vi "nanocal -- nuclear schottky fit V3.vi"() -> ()   [LabVIEW 2020] (continued)
κ0\"-> 0.000000003681  , \"mm1\"-> 0.000000000000  , \"mm2\"-> 0.000000000000  , \"mm3\"-> 0.000000000000  , \"T\"->  0.512000000000  , \"B\"-> 12.000000000000  , \"θ\"-> 90.000000000000  |>   , \r8079 ->   <| \"ζ\"->  0.020568815513  , \"τ1\"-> 0.023045965648  , \"τS\"-> 0.020791387386  , \"τN\"-> 0.002229171297  , \"τC\"-> 0.004427475438  , \"κ0\"-> 0.000000004398  , \"mm1\"-> 0.000000000000  , \"mm2\"-> 0.000000000000  , \"mm3\"-> 0.000000000000  , \"T\"->  0.610000000000  , \"B\"-> 12.000000000000  , \"θ\"-> 90.000000000000  |>   , \r8080 ->   <| \"ζ\"->  0.016548170999  , \"τ1\"-> 0.020108887890  , \"τS\"-> 0.018558394948  , \"τN\"-> 0.001160732495  , \"τC\"-> 0.004746126241  , \"κ0\"-> 0.000000005882  , \"mm1\"-> 0.000000000000  , \"mm2\"-> 0.000000000000  , \"mm3\"-> 0.000000000000  , \"T\"->  0.810000000000  , \"B\"-> 12.000000000000  , \"θ\"-> 90.000000000000  |>   , \r8081 ->   <| \"ζ\"->  0.014495870556  , \"τ1\"-> 0.019990087457  , \"τS\"-> 0.016832201384  , \"τN\"-> 0.000455517238  , \"τC\"-> 0.005555782498  , \"κ0\"-> 0.000000008420  , \"mm1\"-> 0.000000000000  , \"mm2\"-> 0.000000000000  , \"mm3\"-> 0.000000000000  , \"T\"->  1.100000000000  , \"B\"-> 12.000000000000  , \"θ\"-> 90.000000000000  |>   , \r8082 ->   <| \"ζ\"->  0.014043763709  , \"τ1\"-> 0.018292068543  , \"τS\"-> 0.011311396743  , \"τN\"-> 0.000128802259  , \"τC\"-> 0.008087849636  , \"κ0\"-> 0.000000014258  , \"mm1\"-> 0.000000000000  , \"mm2\"-> 0.000000000000  , \"mm3\"-> 0.000000000000  , \"T\"->  1.800000000000  , \"B\"-> 12.000000000000  , \"θ\"-> 90.000000000000  |>   , \r8083 ->   <| \"ζ\"->  0.016187684631  , \"τ1\"-> 0.018325345271  , \"τS\"-> 0.007510087776  , \"τN\"-> 0.000028419157  , \"τC\"-> 0.008115463080  , \"κ0\"-> 0.000000024747  , \"mm1\"-> 0.000000000000  , \"mm2\"-> 0.000000000000  , \"mm3\"-> 0.000000000000  , \"T\"->  3.000000000000  , \"B\"-> 12.000000000000  , \"θ\"-> 90.000000000000  |>   , \r8084 ->   <| \"ζ\"->  0.027897403691  , \"τ1\"-> 0.014639690770  , \"τS\"-> 0.004105291179  , \"τN\"-> 0.000006999171  , \"τC\"-> 0.007414449545  , \"κ0\"-> 0.000000059701  , \"mm1\"-> 0.000000000000  , \"mm2\"-> 0.000000000000  , \"mm3\"-> 0.000000000000  , \"T\"->  5.700000000000  , \"B\"-> 12.000000000000  , \"θ\"-> 90.000000000000  |>   , \r8094 ->   <| \"ζ\"->  0.000000000000  , \"τ1\"-> 0.000000000000  , \"τS\"-> 0.000000000000  , \"τN\"-> 0.000000000000  , \"τC\"-> 0.000000000000  , \"κ0\"-> 0.000000000000  , \"mm1\"-> 0.000000000000  , \"mm2\"-> 0.000000000000  , \"mm3\"-> 0.000000000000  , \"T\"->  0.300000000000  , \"B\"-> 6.000000000000  , \"θ\"-> 90.000000000000  |>   , \r8095 ->   <| \"ζ\"->  0.132901556203  , \"τ1\"-> 0.022795175616  , \"τS\"-> 0.082481385864  , \"τN\"-> 0.041432545456  , \"τC\"-> 0.001408424074  , \"κ0\"-> 0.000000001182  , \"mm1\"-> 0.000000000000  , \"mm2\"-> 0.000000000000  , \"mm3\"-> 0.000000000000  , \"T\"->  0.197000000000  , \"B\"-> 6.000000000000  , \"θ\"-> 90.000000000000  |>   , \r8098 ->   <| \"ζ\"->  0.000000000000  , \"τ1\"-> 0.000000000000  , \"τS\"-> 0.000000000000  , \"τN\"-> 0.000000000000  , \"τC\"-> 0.000000000000  , \"κ0\"-> 0.000000000000  , \"mm1\"-> 0.000000000000  , \"mm2\"-> 0.000000000000  , \"mm3\"-> 0.000000000000  , \"T\"->  0.148000000000  , \"B\"-> 6.000000000000  , \"θ\"-> 90.000000000000  |>   , \r8099 ->   <| \"ζ\"->  0.132534999612  , \"τ1\"-> 0.042581417401  , \"τS\"-> 0.054103824371  , \"τN\"-> 0.072163013930  , \"τC\"-> 0.001421040158  , \"κ0\"-> 0.000000001190  , \"mm1\"-> 0.000000000000  , \"mm2\"-> 0.000000000000  , \"mm3\"-> 0.000000000000  , \"T\"->  0.197000000000  , \"B\"-> 9.000000000000  , \"θ\"-> 90.000000000000  |>   , \r8100 ->   <| \"ζ\"->  0.124414912597  , \"τ1\"-> 0.052685716706  , \"τS\"-> 0.041788480794  , \"τN\"-> 0.092820346766  , \"τC\"-> 0.001183564004  , \"κ0\"-> 0.000000001217  , \"mm1\"-> 0.000000000000  , \"mm2\"-> 0.000000000000  , \"mm3\"-> 0.000000000000  , \"T\"->  0.197000000000  , \"B\"-> 11.000000000000  , \"θ\"-> 90.000000000000  |>   , \r8101 ->   <| \"ζ\"->  0.130083148284  , \"τ1\"-> 0.046211117525  , \"τS\"-> 0.046173592526  , \"τN\"-> 0.081942172735  , \"τC\"-> 0.001380184863  , \"κ0\"-> 0.000000001209  , \"mm1\"-> 0.000000000000  , \"mm2\"-> 0.000000000000  , \"mm3\"-> 0.000000000000  , \"T\"->  0.197000000000  , \"B\"-> 10.000000000000  , \"θ\"-> 90.000000000000  |>   , \r8102 ->   <| \"ζ\"->  0.126440702434  , \"τ1\"-> 0.034118036572  , \"τS\"-> 0.060921114440  , \"τN\"-> 0.059832148427  , \"τC\"-> 0.001404471084  , \"κ0\"-> 0.000000001199  , \"mm1\"-> 0.000000000000  , \"mm2\"-> 0.000000000000  , \"mm3\"-> 0.000000000000  , \"T\"->  0.197000000000  , \"B\"-> 8.000000000000  , \"θ\"-> 90.000000000000  |>   , \r8103 ->   <| \"ζ\"->  0.131383255045  , \"τ1\"-> 0.026827335842  , \"τS\"-> 0.071725959535  , \"τN\"-> 0.047510049318  , \"τC\"-> 0.001407613780  , \"κ0\"-> 0.000000001187  , \"mm1\"-> 0.000000000000  , \"mm2\"-> 0.000000000000  , \"mm3\"-> 0.000000000000  , \"T\"->  0.197000000000  , \"B\"-> 7.000000000000  , \"θ\"-> 90.000000000000  |>   , \r8104 ->   <| \"ζ\"->  0.125455081262  , \"τ1\"-> 0.021777951907  , \"τS\"-> 0.089086097551  , \"τN\"-> 0.033580911935  , \"τC\"-> 0.001437991682  , \"κ0\"-> 0.000000001167  , \"mm1\"-> 0.000000000000  , \"mm2\"-> 0.000000000000  , \"mm3\"-> 0.000000000000  , \"T\"->  0.197000000000  , \"B\"-> 5.000000000000  , \"θ\"-> 90.000000000000  |>   , \r8105 ->   <| \"ζ\"->  0.101804363109  , \"τ1\"-> 0.031947692776  , \"τS\"-> 0.014125667853  , \"τN\"-> 0.006009042128  , \"τC\"-> 0.002323789932  , \"κ0\"-> 0.000000001168  , \"mm1\"-> 0.000000000000  , \"mm2\"-> 0.000000000000  , \"mm3\"-> 0.000000000000  , \"T\"->  0.197000000000  , \"B\"-> 0.000000000000  , \"θ\"-> 90.000000000000  |>   , \r8106 ->   <| \"ζ\"->  0.000000000000  , \"τ1\"-> 0.000000000000  , \"τS\"-> 0.000000000000  , \"τN\"-> 0.000000000000  , \"τC\"-> 0.000000000000  , \"κ0\"-> 0.000000000000  , \"mm1\"-> 0.000000000000  , \"mm2\"-> 0.000000000000  , \"mm3\"-> 0.000000000000  , \"T\"->  1.550000000000  , \"B\"-> 0.000000000000  , \"θ\"-> 90.000000000000  |>   , \r8107 ->   <| \"ζ\"->  0.000000000000  , \"τ1\"-> 0.000000000000  , \"τS\"-> 0.000000000000  , \"τN\"-> 0.000000000000  , \"τC\"-> 0.000000000000  , \"κ0\"-> 0.000000000000  , \"mm1\"-> 0.000000000000  , \"mm2\"-> 0.000000000000  , \"mm3\"-> 0.000000000000  , \"T\"->  1.000000000000  , \"B\"-> 0.000000000000  , \"θ\"-> 90.000000000000  |>   , \r8108 ->   <| \"ζ\"->  0.000000000000  , \"τ1\"-> 0.000000000000  , \"τS\"-> 0.000000000000  , \"τN\"-> 0.000000000000  , \"τC\"-> 0.000000000000  , \"κ0\"-> 0.000000000000  , \"mm1\"-> 0.000000000000  , \"mm2\"-> 0.000000000000  , \"mm3\"-> 0.000000000000  , \"T\"->  0.670000000000  , \"B\"-> 0.000000000000  , \"θ\"-> 90.000000000000  |>   , \r8110 ->   <| \"ζ\"->  0.162585495535  , \"τ1\"-> 0.037883389730  , \"τS\"-> 0.086562863191  , \"τN\"-> 0.241872534356  , \"τC\"-> 0.001506143871  , \"κ0\"-> 0.000000000791  , \"mm1\"-> 0.000000000000  , \"mm2\"-> 0.000000000000  , \"mm3\"-> 0.000000000000  , \"T\"->  0.160000000000  , \"B\"-> 12.000000000000  , \"θ\"-> 30.000000000000  |>   , \r8112 ->   <| \"ζ\"->  0.156472219566  , \"τ1\"-> 0.031017925061  , \"τS\"-> 0.080872234530  , \"τN\"-> 0.219381306397  , \"τC\"-> 0.001437792153  , \"κ0\"-> 0.000000000867  , \"mm1\"-> 0.000000000000  , \"mm2\"-> 0.000000000000  , \"mm3\"-> 0.000000000000  , \"T\"->  0.170000000000  , \"B\"-> 12.000000000000  , \"θ\"-> 30.000000000000  |>   , \r8113 ->   <| \"ζ\"->  0.211545693132  , \"τ1\"-> 0.029106147473  , \"τS\"-> 0.094475691604  , \"τN\"-> 0.369151052631  , \"τC\"-> 0.001396700790  , \"κ0\"-> 0.000000000537  , \"mm1\"-> 0.000000000000  , \"mm2\"-> 0.000000000000  , \"mm3\"-> 0.000000000000  , \"T\"->  0.140000000000  , \"B\"-> 12.000000000000  , \"θ\"-> 30.000000000000  |>   , \r8114 ->   <| \"ζ\"->  0.128615765969  , \"τ1\"-> 0.032665502211  , \"τS\"-> 0.082694869013  , \"τN\"-> 0.105788373632  , \"τC\"-> 0.001439686784  , \"κ0\"-> 0.000000001168  , \"mm1\"-> 0.000000000000  , \"mm2\"-> 0.000000000000  , \"mm3\"-> 0.000000000000  , \"T\"->  0.200000000000  , \"B\"-> 12.000000000000  , \"θ\"-> 30.000000000000  |>   , \r8115 ->   <| \"ζ\"->  0.072634365939  , \"τ1\"-> 0.028637109000  , \"τS\"-> 0.065061142288  , \"τN\"-> 0.040304243071  , \"τC\"-> 0.001622979999  , \"κ0\"-> 0.000000001498  , \"mm1\"-> 0.000000000000  , \"mm2\"-> 0.000000000000  , \"mm3\"-> 0.000000000000  , \"T\"->  0.250000000000  , \"B\"-> 12.000000000000  , \"θ\"-> 30.000000000000  |>   , \r8116 ->   <| \"ζ\"->  0.050663808076  , \"τ1\"-> 0.024940898568  , \"τS\"-> 0.056803871413  , \"τN\"-> 0.018856862265  , \"τC\"-> 0.002133501904  , \"κ0\"-> 0.000000001888  , \"mm1\"-> 0.000000000000  , \"mm2\"-> 0.000000000000  , \"mm3\"-> 0.000000000000  , \"T\"->  0.300000000000  , \"B\"-> 12.000000000000  , \"θ\"-> 30.000000000000  |>   , \r8117 ->   <| \"ζ\"->  0.036420486357  , \"τ1\"-> 0.020986681106  , \"τS\"-> 0.049149577509  , \"τN\"-> 0.011109585503  , \"τC\"-> 0.002819780093  , \"κ0\"-> 0.000000002299  , \"mm1\"-> 0.000000000000  , \"mm2\"-> 0.000000000000  , \"mm3\"-> 0.000000000000  , \"T\"->  0.360000000000  , \"B\"-> 12.000000000000  , \"θ\"-> 30.000000000000  |>   , \r8118 ->   <| \"ζ\"->  0.028468689077  , \"τ1\"-> 0.020220821810  , \"τS\"-> 0.043529484347  , \"τN\"-> 0.005653540941  , \"τC\"-> 0.003150537442  , \"κ0\"-> 0.000000002855  , \"mm1\"-> 0.000000000000  , \"mm2\"-> 0.000000000000  , \"mm3\"-> 0.000000000000  , \"T\"->  0.430000000000  , \"B\"-> 12.000000000000  , \"θ\"-> 30.000000000000  |>   , \r8119 ->   <| \"ζ\"->  0.021116250068  , \"τ1\"-> 0.020669239851  , \"τS\"-> 0.037941648749  , \"τN\"-> 0.003221866945  , \"τC\"-> 0.003619427775  , \"κ0\"-> 0.000000003553  , \"mm1\"-> 0.000000000000  , \"mm2\"-> 0.000000000000  , \"mm3\"-> 0.000000000000  , \"T\"->  0.530000000000  , \"B\"-> 12.000000000000  , \"θ\"-> 30.000000000000  |>   , \r8120 ->   <| \"ζ\"->  0.016892016292  , \"τ1\"-> 0.020344757415  , \"τS\"-> 0.033845756966  , \"τN\"-> 0.001946817417  , \"τC\"-> 0.004013762913  , \"κ0\"-> 0.000000004252  , \"mm1\"-> 0.000000000000  , \"mm2\"-> 0.000000000000  , \"mm3\"-> 0.000000000000  , \"T\"->  0.620000000000  , \"B\"-> 12.000000000000  , \"θ\"-> 30.000000000000  |>   , \r8121 ->   <| \"ζ\"->  0.013460153434  , \"τ1\"-> 0.020684726260  , \"τS\"-> 0.027140346721  , \"τN\"-> 0.000960302406  , \"τC\"-> 0.004517434882  , \"κ0\"-> 0.000000005889  , \"mm1\"-> 0.000000000000  , \"mm2\"-> 0.000000000000  , \"mm3\"-> 0.000000000000  , \"T\"->  0.830000000000  , \"B\"-> 12.000000000000  , \"θ\"-> 30.000000000000  |>   , \r8122 ->   <| \"ζ\"->  0.010912011148  , \"τ1\"-> 0.020760977312  , \"τS\"-> 0.021106239637  , \"τN\"-> 0.000452316988  , \"τC\"-> 0.005003723454  , \"κ0\"-> 0.000000008194  , \"mm1\"-> 0.000000000000  , \"mm2\"-> 0.000000000000  , \"mm3\"-> 0.000000000000  , \"T\"->  1.130000000000  , \"B\"-> 12.000000000000  , \"θ\"-> 30.000000000000  |>   , \r8123 ->   <| \"ζ\"->  0.009772435939  , \"τ1\"-> 0.020827345370  , \"τS\"-> 0.013809334085  , \"τN\"-> 0.000168485133  , \"τC\"-> 0.005555066716  , \"κ0\"-> 0.000000013930  , \"mm1\"-> 0.000000000000  , \"mm2\"-> 0.000000000000  , \"mm3\"-> 0.000000000000  , \"T\"->  1.900000000000  , \"B\"-> 12.000000000000  , \"θ\"-> 30.000000000000  |>   , \r8124 ->   <| \"ζ\"->  0.010111127240  , \"τ1\"-> 0.020788755574  , \"τS\"-> 0.009968978424  , \"τN\"-> 0.000077788811  , \"τC\"-> 0.004598584548  , \"κ0\"-> 0.000000024346  , \"mm1\"-> 0.000000000000  , \"mm2\"-> 0.000000000000  , \"mm3\"-> 0.000000000000  , \"T\"->  3.100000000000  , \"B\"-> 12.000000000000  , \"θ\"-> 30.000000000000  |>   , \r40047 ->   <| \"ζ\"->  0.020744689680  , \"τ1\"-> 0.017944253087  , \"τS\"-> 0.003548154619  , \"τN\"-> 0.000036329906  , \"τC\"-> 0.004738266852  , \"κ0\"-> 0.000000058027  , \"mm1\"-> 0.000000000000  , \"mm2\"-> 0.000000000000  , \"mm3\"-> 0.000000000000  , \"T\"->  19.600000000000  , \"B\"-> 12.000000000000  , \"θ\"-> 60.000000000000  |>   , \r40049 ->   <| \"ζ\"->  0.334519022578  , \"τ1\"-> 0.071617660141  , \"τS\"-> 0.066230384072  , \"τN\"-> 0.374518999658  , \"τC\"-> 0.002158821958  , \"κ0\"-> 0.000000000405  , \"mm1\"-> 0.000000000000  , \"mm2\"-> 0.000000000000  , \"mm3\"-> 0.000000000000  , \"T\"->  0.129000000000  , \"B\"-> 12.000000000000  , \"θ\"-> 60.000000000000  |>   , \r40125 ->   <| \"ζ\"->  0.295520923520  , \"τ1\"-> 0.054772440405  , \"τS\"-> 0.071814005451  , \"τN\"-> 0.249593767169  , \"τC\"-> 0.001103632155  , \"κ0\"-> 0.000000000625  , \"mm1\"-> 0.000000000000  , \"mm2\"-> 0.000000000000  , \"mm3\"-> 0.000000000000  , \"T\"->  0.157000000000  , \"B\"-> 12.000000000000  , \"θ\"-> 45.000000000000  |>   , \r40126 ->   <| \"ζ\"->  0.523545279740  , \"τ1\"-> 0.065613539167  , \"τS\"-> 0.100000000000  , \"τN\"-> 0.424083114177  , \"τC\"-> 0.000911255863  , \"κ0\"-> 0.000000000418  , \"mm1\"-> 0.000000000000  , \"mm2\"-> 0.000000000000  , \"mm3\"-> 0.000000000000  , \"T\"->  0.120000000000  , \"B\"-> 12.000000000000  , \"θ\"-> 45.000000000000  |>   , \r40127 ->   <| \"ζ\"->  0.273742116471  , \"τ1\"-> 0.052262909995  , \"τS\"-> 0.060554036646  , \"τN\"-> 0.154269705680  , \"τC\"-> 0.001074144337  , \"κ0\"-> 0.000000000753  , \"mm1\"-> 0.000000000000  , \"mm2\"-> 0.000000000000  , \"mm3\"-> 0.000000000000  , \"T\"->  0.170000000000  , \"B\"-> 12.000000000000  , \"θ\"-> 45.000000000000  |>   , \r40128 ->   <| \"ζ\"->  0.215688135788  , \"τ1\"-> 0.043710888546  , \"τS\"-> 0.044756474141  , \"τN\"-> 0.090222547904  , \"τC\"-> 0.001049781785  , \"κ0\"-> 0.000000001047  , \"mm1\"-> 0.000000000000  , \"mm2\"-> 0.000000000000  , \"mm3\"-> 0.000000000000  , \"T\"->  0.200000000000  , \"B\"-> 12.000000000000  , \"θ\"-> 45.000000000000  |>   , \r40129 ->   <| \"ζ\"->  0.118583992968  , \"τ1\"-> 0.035232851003  , \"τS\"-> 0.037458022816  , \"τN\"-> 0.033724509363  , \"τC\"-> 0.001440922263  , \"κ0\"-> 0.000000001360  , \"mm1\"-> 0.000000000000  , \"mm2\"-> 0.000000000000  , \"mm3\"-> 0.000000000000  , \"T\"->  0.255000000000  , \"B\"-> 12.000000000000  , \"θ\"-> 45.000000000000  |>   , \r40130 ->   <| \"ζ\"->  0.085152769414  , \"τ1\"-> 0.029001116263  , \"τS\"-> 0.032604663993  , \"τN\"-> 0.016878763935  , \"τC\"-> 0.001443524845  , \"κ0\"-> 0.000000001728  , \"mm1\"-> 0.000000000000  , \"mm2\"-> 0.000000000000  , \"mm3\"-> 0.000000000000  , \"T\"->  0.300000000000  , \"B\"-> 12.000000000000  , \"θ\"-> 45.000000000000  |>   , \r40131 ->   <| \"ζ\"->  0.061011838044  , \"τ1\"-> 0.025440548989  , \"τS\"-> 0.030028053978  , \"τN\"-> 0.010140731955  , \"τC\"-> 0.001895079687  , \"κ0\"-> 0.000000002115  , \"mm1\"-> 0.000000000000  , \"mm2\"-> 0.000000000000  , \"mm3\"-> 0.000000000000  , \"T\"->  0.360000000000  , \"B\"-> 12.000000000000  , \"θ\"-> 45.000000000000  |>   , \r40132 ->   <| \"ζ\"->  0.046686299518  , \"τ1\"-> 0.021011215626  , \"τS\"-> 0.027633142317  , \"τN\"-> 0.005348477555  , \"τC\"-> 0.002098477650  , \"κ0\"-> 0.000000002635  , \"mm1\"-> 0.000000000000  , \"mm2\"-> 0.000000000000  , \"mm3\"-> 0.000000000000  , \"T\"->  0.430000000000  , \"B\"-> 12.000000000000  , \"θ\"-> 45.000000000000  |>   , \r40133 ->   <| \"ζ\"->  0.035204330012  , \"τ1\"-> 0.021011523093  , \"τS\"-> 0.025247316079  , \"τN\"-> 0.002718647875  , \"τC\"-> 0.003091727575  , \"κ0\"-> 0.000000003296  , \"mm1\"-> 0.000000000000  , \"mm2\"-> 0.000000000000  , \"mm3\"-> 0.000000000000  , \"T\"->  0.530000000000  , \"B\"-> 12.000000000000  , \"θ\"-> 45.000000000000  |>   , \r40134 ->   <| \"ζ\"->  0.030862035723  , \"τ1\"-> 0.019328530751  , \"τS\"-> 0.023568572597  , \"τN\"-> 0.001701966614  , \"τC\"-> 0.003453790534  , \"κ0\"-> 0.000000003906  , \"mm1\"-> 0.000000000000  , \"mm2\"-> 0.000000000000  , \"mm3\"-> 0.000000000000  , \"T\"->  0.620000000000  , \"B\"-> 12.000000000000  , \"θ\"-> 45.000000000000  |>   , \r40135 ->   <| \"ζ\"->  0.023591124045  , \"τ1\"-> 0.014910006225  , \"τS\"-> 0.019342950404  , \"τN\"-> 0.000752972387  , \"τC\"-> 0.004900413232  , \"κ0\"-> 0.000000005453  , \"mm1\"-> 0.000000000000  , \"mm2\"-> 0.000000000000  , \"mm3\"-> 0.000000000000  , \"T\"->  0.830000000000  , \"B\"-> 12.000000000000  , \"θ\"-> 45.000000000000  |>   , \r40136 ->   <| \"ζ\"->  0.020215154826  , \"τ1\"-> 0.014105227254  , \"τS\"-> 0.015660924043  , \"τN\"-> 0.000525137036  , \"τC\"-> 0.005447728357  , \"κ0\"-> 0.000000007594  , \"mm1\"-> 0.000000000000  , \"mm2\"-> 0.000000000000  , \"mm3\"-> 0.000000000000  , \"T\"->  1.130000000000  , \"B\"-> 12.000000000000  , \"θ\"-> 45.000000000000  |>   , \r40137 ->   <| \"ζ\"->  0.018090572724  , \"τ1\"-> 0.013314780956  , \"τS\"-> 0.010820835010  , \"τN\"-> 0.000265552167  , \"τC\"-> 0.005393540417  , \"κ0\"-> 0.000000013100  , \"mm1\"-> 0.000000000000  , \"mm2\"-> 0.000000000000  , \"mm3\"-> 0.000000000000  , \"T\"->  1.900000000000  , \"B\"-> 12.000000000000  , \"θ\"-> 45.000000000000  |>   , \r40138 ->   <| \"ζ\"->  0.019438138135  , \"τ1\"-> 0.013521019406  , \"τS\"-> 0.007253169401  , \"τN\"-> 0.000154824830  , \"τC\"-> 0.004746579385  , \"κ0\"-> 0.000000023466  , \"mm1\"-> 0.000000000000  , \"mm2\"-> 0.000000000000  , \"mm3\"-> 0.000000000000  , \"T\"->  3.100000000000  , \"B\"-> 12.000000000000  , \"θ\"-> 45.000000000000  |>   , \r40139 ->   <| \"ζ\"->  0.018573189054  , \"τ1\"-> 0.013304612245  , \"τS\"-> 0.003723860844  , \"τN\"-> 0.000084829442  , \"τC\"-> 0.004309703632  , \"κ0\"-> 0.000000058362  , \"mm1\"-> 0.000000000000  , \"mm2\"-> 0.000000000000  , \"mm3\"-> 0.000000000000  , \"T\"->  5.700000000000  , \"B\"-> 12.000000000000  , \"θ\"-> 45.000000000000  |>   , \r80047 ->   <| \"ζ\"->  0.000000000000  , \"τ1\"-> 0.000000000000  , \"τS\"-> 0.000000000000  , \"τN\"-> 0.000000000000  , \"τC\"-> 0.000000000000  , \"κ0\"-> 0.000000000000  , \"mm1\"-> 0.000000000000  , \"mm2\"-> 0.000000000000  , \"mm3\"-> 0.000000000000  , \"T\"->  19.600000000000  , \"B\"-> 12.000000000000  , \"θ\"-> 60.000000000000  |>   , \r80049 ->   <| \"ζ\"->  0.206128000000  , \"τ1\"-> 0.061001000000  , \"τS\"-> 0.056065000000  , \"τN\"-> 0.442324169403  , \"τC\"-> 0.001917000000  , \"κ0\"-> 0.000000000541  , \"mm1\"-> 0.000000000000  , \"mm2\"-> 0.000000000000  , \"mm3\"-> 0.000000000000  , \"T\"->  0.129000000000  , \"B\"-> 12.000000000000  , \"θ\"-> 60.000000000000  |>   , \r80125 ->   <| \"ζ\"->  0.000000000000  , \"τ1\"-> 0.000000000000  , \"τS\"-> 0.000000000000  , \"τN\"-> 0.000000000000  , \"τC\"-> 0.000000000000  , \"κ0\"-> 0.000000000000  , \"mm1\"-> 0.000000000000  , \"mm2\"-> 0.000000000000  , \"mm3\"-> 0.000000000000  , \"T\"->  0.157000000000  , \"B\"-> 12.000000000000  , \"θ\"-> 45.000000000000  |>   , \r80126 ->   <| \"ζ\"->  0.000000000000  , \"τ1\"-> 0.000000000000  , \"τS\"-> 0.000000000000  , \"τN\"-> 0.000000000000  , \"τC\"-> 0.000000000000  , \"κ0\"-> 0.000000000000  , \"mm1\"-> 0.000000000000  , \"mm2\"-> 0.000000000000  , \"mm3\"-> 0.000000000000  , \"T\"->  0.120000000000  , \"B\"-> 12.000000000000  , \"θ\"-> 45.000000000000  |>   , \r80127 ->   <| \"ζ\"->  0.000000000000  , \"τ1\"-> 0.000000000000  , \"τS\"-> 0.000000000000  , \"τN\"-> 0.000000000000  , \"τC\"-> 0.000000000000  , \"κ0\"-> 0.000000000000  , \"mm1\"-> 0.000000000000  , \"mm2\"-> 0.000000000000  , \"mm3\"-> 0.000000000000  , \"T\"->  0.170000000000  , \"B\"-> 12.000000000000  , \"θ\"-> 45.000000000000  |>   , \r80128 ->   <| \"ζ\"->  0.000000000000  , \"τ1\"-> 0.000000000000  , \"τS\"-> 0.000000000000  , \"τN\"-> 0.000000000000  , \"τC\"-> 0.000000000000  , \"κ0\"-> 0.000000000000  , \"mm1\"-> 0.000000000000  , \"mm2\"-> 0.000000000000  , \"mm3\"-> 0.000000000000  , \"T\"->  0.200000000000  , \"B\"-> 12.000000000000  , \"θ\"-> 45.000000000000  |>   , \r80129 ->   <| \"ζ\"->  0.000000000000  , \"τ1\"-> 0.000000000000  , \"τS\"-> 0.000000000000  , \"τN\"-> 0.000000000000  , \"τC\"-> 0.000000000000  , \"κ0\"-> 0.000000000000  , \"mm1\"-> 0.000000000000  , \"mm2\"-> 0.000000000000  , \"mm3\"-> 0.000000000000  , \"T\"->  0.255000000000  , \"B\"-> 12.000000000000  , \"θ\"-> 45.000000000000  |>   , \r80130 ->   <| \"ζ\"->  0.000000000000  , \"τ1\"-> 0.000000000000  , \"τS\"-> 0.000000000000  , \"τN\"-> 0.000000000000  , \"τC\"-> 0.000000000000  , \"κ0\"-> 0.000000000000  , \"mm1\"-> 0.000000000000  , \"mm2\"-> 0.000000000000  , \"mm3\"-> 0.000000000000  , \"T\"->  0.300000000000  , \"B\"-> 12.000000000000  , \"θ\"-> 45.000000000000  |>   , \r80131 ->   <| \"ζ\"->  0.000000000000  , \"τ1\"-> 0.000000000000  , \"τS\"-> 0.000000000000  , \"τN\"-> 0.000000000000  , \"τC\"-> 0.000000000000  , \"κ0\"-> 0.000000000000  , \"mm1\"-> 0.000000000000  , \"mm2\"-> 0.000000000000  , \"mm3\"-> 0.000000000000  , \"T\"->  0.360000000000  , \"B\"-> 12.000000000000  , \"θ\"-> 45.000000000000  |>   , \r80132 ->   <| \"ζ\"->  0.000000000000  , \"τ1\"-> 0.000000000000  , \"τS\"-> 0.000000000000  , \"τN\"-> 0.000000000000  , \"τC\"-> 0.000000000000  , \"κ0\"-> 0.000000000000  , \"mm1\"-> 0.000000000000  , \"mm2\"-> 0.000000000000  , \"mm3\"-> 0.000000000000  , \"T\"->  0.430000000000  , \"B\"-> 12.000000000000  , \"θ\"-> 45.000000000000  |>   , \r80133 ->   <| \"ζ\"->  0.000000000000  , \"τ1\"-> 0.000000000000  , \"τS\"-> 0.000000000000  , \"τN\"-> 0.000000000000  , \"τC\"-> 0.000000000000  , \"κ0\"-> 0.000000000000  , \"mm1\"-> 0.000000000000  , \"mm2\"-> 0.000000000000  , \"mm3\"-> 0.000000000000  , \"T\"->  0.530000000000  , \"B\"-> 12.000000000000  , \"θ\"-> 45.000000000000  |>   , \r80134 ->   <| \"ζ\"->  0.000000000000  , \"τ1\"-> 0.000000000000  , \"τS\"-> 0.000000000000  , \"τN\"-> 0.000000000000  , \"τC\"-> 0.000000000000  , \"κ0\"-> 0.000000000000  , \"mm1\"-> 0.000000000000  , \"mm2\"-> 0.000000000000  , \"mm3\"-> 0.000000000000  , \"T\"->  0.620000000000  , \"B\"-> 12.000000000000  , \"θ\"-> 45.000000000000  |>   , \r80135 ->   <| \"ζ\"->  0.000000000000  , \"τ1\"-> 0.000000000000  , \"τS\"-> 0.000000000000  , \"τN\"-> 0.000000000000  , \"τC\"-> 0.000000000000  , \"κ0\"-> 0.000000000000  , \"mm1\"-> 0.000000000000  , \"mm2\"-> 0.000000000000  , \"mm3\"-> 0.000000000000  , \"T\"->  0.830000000000  , \"B\"-> 12.000000000000  , \"θ\"-> 45.000000000000  |>   , \r80136 ->   <| \"ζ\"->  0.000000000000  , \"τ1\"-> 0.000000000000  , \"τS\"-> 0.000000000000  , \"τN\"-> 0.000000000000  , \"τC\"-> 0.000000000000  , \"κ0\"-> 0.000000000000  , \"mm1\"-> 0.000000000000  , \"mm2\"-> 0.000000000000  , \"mm3\"-> 0.000000000000  , \"T\"->  1.130000000000  , \"B\"-> 12.000000000000  , \"θ\"-> 45.000000000000  |>   , \r80137 ->   <| \"ζ\"->  0.000000000000  , \"τ1\"-> 0.000000000000  , \"τS\"-> 0.000000000000  , \"τN\"-> 0.000000000000  , \"τC\"-> 0.000000000000  , \"κ0\"-> 0.000000000000  , \"mm1\"-> 0.000000000000  , \"mm2\"-> 0.000000000000  , \"mm3\"-> 0.000000000000  , \"T\"->  1.900000000000  , \"B\"-> 12.000000000000  , \"θ\"-> 45.000000000000  |>   , \r80138 ->   <| \"ζ\"->  0.000000000000  , \"τ1\"-> 0.000000000000  , \"τS\"-> 0.000000000000  , \"τN\"-> 0.000000000000  , \"τC\"-> 0.000000000000  , \"κ0\"-> 0.000000000000  , \"mm1\"-> 0.000000000000  , \"mm2\"-> 0.000000000000  , \"mm3\"-> 0.000000000000  , \"T\"->  3.100000000000  , \"B\"-> 12.000000000000  , \"θ\"-> 45.000000000000  |>   , \r80139 ->   <| \"ζ\"->  0.000000000000  , \"τ1\"-> 0.000000000000  , \"τS\"-> 0.000000000000  , \"τN\"-> 0.000000000000  , \"τC\"-> 0.000000000000  , \"κ0\"-> 0.000000000000  , \"mm1\"-> 0.000000000000  , \"mm2\"-> 0.000000000000  , \"mm3\"-> 0.000000000000  , \"T\"->  5.700000000000  , \"B\"-> 12.000000000000  , \"θ\"-> 45.000000000000  |>   , \r"
  in  "Math --> string OUT!":bool
  in  "string IN  --> Math!":bool
  in  "file pattern":string="CeCoIn5_*_labview_.dat"
  in  "folder":path=path "/opt/new/Dropbox/shared_AkashAndreas/paper-CeCoIn5/dataset--changeT--12T--0deg--60deg--90deg"
  in  "filenames":u16(ring)=29 caption="files" items=["CeCoIn5_2nd_8047_12T_sam_0.12K_0deg_changeT_fsweep_labview_.dat", "CeCoIn5_2nd_8071_12T_sam_0.120K_90deg_changeT_fsweep_labview_.dat", "CeCoIn5_4th___40126__(040)__C(f)_12T_0.120K_45deg_changeT_ref_fromraw__labview_.dat", "CeCoIn5_4th___80126__(040)__C(f)_12T_0.120K_45deg_changeT_sam_fromraw__labview_.dat", "CeCoIn5_3rd_4026_ref_12T_0.127K_60deg_changeT_fsweep_labview_.dat", "CeCoIn5_3rd_8026_sam_12T_0.127K_60deg_changeT_fsweep_labview_.dat", "CeCoIn5_3rd_40049_ref_12T_0.129K_60deg_changeT_fsweep_labview_.dat", "CeCoIn5_3rd_80049_sam_12T_0.129K_60deg_changeT_fsweep_labview_.dat", "CeCoIn5_2nd_4047_12T_ref_0.14K_0deg_changeT_fsweep_labview_.dat", "CeCoIn5_2nd_4071_12T_ref_0.14K_90deg_changeT_fsweep_labview_.dat", "CeCoIn5_4th_4113_ref_12T_0.14K_30deg_changeT_fsweep_labview_.dat", "CeCoIn5_4th_8113_sam_12T_0.14K_30deg_changeT_fsweep_labview_.dat", "CeCoIn5_2nd_4098_6T_0.148K_90deg_ref_changeB_fsweep_labview_.dat", "CeCoIn5_2nd_8048_12T_sam_0.148K_0deg_changeT_fsweep_labview_.dat", "CeCoIn5_2nd_8072_12T_sam_0.148K_90deg_changeT_fsweep_labview_.dat", "CeCoIn5_2nd_8098_6T_0.148K_90deg_sam_changeB_fsweep_labview_.dat", "CeCoIn5_3rd_4027_ref_12T_0.15K_60deg_changeT_fsweep_labview_.dat", "CeCoIn5_3rd_8027_sam_12T_0.15K_60deg_changeT_fsweep_labview_.dat", "CeCoIn5_4th___40125__(039)__C(f)_12T_0.157K_45deg _changeT_ref_fromraw__labview_.dat", "CeCoIn5_4th___80125__(039)__C(f)_12T_0.157K_45deg _changeT_sam_fromraw__labview_.dat", "CeCoIn5_4th_4110_ref_12T_0.16K_30deg_changeT_fsweep_labview_.dat", "CeCoIn5_4th_8110_sam_12T_0.16K_30deg_changeT_fsweep_labview_.dat", "CeCoIn5_2nd_4048_12T_ref_0.17K_0deg_changeT_fsweep_labview_.dat", "CeCoIn5_4th_4112_ref_12T_0.17K_30deg_changeT_fsweep_labview_.dat", "CeCoIn5_4th_8112_sam_12T_0.17K_30deg_changeT_fsweep_labview_.dat", "CeCoIn5_4th___40127__(041)__C(f)_12T_0.170K_45deg_changeT_ref_fromraw__labview_.dat", "CeCoIn5_4th___80127__(041)__C(f)_12T_0.170K_45deg_changeT_sam_fromraw__labview_.dat", "CeCoIn5_3rd_4028_ref_12T_0.179K_60deg_changeT_fsweep_labview_.dat", "CeCoIn5_3rd_8028_sam_12T_0.179K_60deg_changeT_fsweep_labview_.dat", "CeCoIn5_2nd_8049_12T_sam_0.179K_0deg_changeT_fsweep_labview_.dat", "CeCoIn5_2nd_8070_12T_sam_0.179K_90deg_changeT_fsweep_labview_.dat", "CeCoIn5_2nd_4072_12T_ref_0.18K_90deg_changeT_fsweep_labview_.dat", "CeCoIn5_2nd_4095_6T_0.197K_90deg_ref_changeB_fsweep_labview_.dat", "CeCoIn5_2nd_4099_9T_0.197K_90deg_ref_changeB_fsweep_labview_.dat", "CeCoIn5_2nd_4100_11T_0.197K_90deg_ref_changeB_fsweep_labview_.dat", "CeCoIn5_2nd_4101_10T_0.197K_90deg_ref_changeB_fsweep_labview_.dat", "CeCoIn5_2nd_4102_8T_0.197K_90deg_ref_changeB_fsweep_labview_.dat", "CeCoIn5_2nd_4103_7T_0.197K_90deg_ref_changeB_fsweep_labview_.dat", "CeCoIn5_2nd_4104_5T_0.197K_90deg_ref_changeB_fsweep_labview_.dat", "CeCoIn5_2nd_4105_0T_0.197K_90deg_ref_changeB_fsweep_labview_.dat", "CeCoIn5_2nd_8050_12T_sam_0.197K_0deg_changeT_fsweep_labview_.dat", "CeCoIn5_2nd_8073_12T_sam_0.197K_90deg_changeT_fsweep_labview_.dat", "CeCoIn5_2nd_8095_6T_0.197K_90deg_sam_changeB_fsweep_labview_.dat", "CeCoIn5_2nd_8099_9T_0.197K_90deg_sam_changeB_fsweep_labview_.dat", "CeCoIn5_2nd_8100_11T_0.197K_90deg_sam_changeB_fsweep_labview_.dat", "CeCoIn5_2nd_8101_10T_0.197K_90deg_sam_changeB_fsweep_labview_.dat", "CeCoIn5_2nd_8102_8T_0.197K_90deg_sam_changeB_fsweep_labview_.dat", "CeCoIn5_2nd_8103_7T_0.197K_90deg_sam_changeB_fsweep_labview_.dat", "CeCoIn5_2nd_8104_5T_0.197K_90deg_sam_changeB_fsweep_labview_.dat", "CeCoIn5_2nd_8105_0T_0.197K_90deg_sam_changeB_fsweep_labview_.dat", "CeCoIn5_3rd_4029_ref_12T_0.20K_60deg_changeT_fsweep_labview_.dat", "CeCoIn5_2nd_4049_12T_ref_0.20K_0deg_changeT_fsweep_labview_.dat", "CeCoIn5_2nd_4070_12T_ref_0.20K_90deg_changeT_fsweep_labview_.dat", "CeCoIn5_4th_4114_ref_12T_0.20K_30deg_changeT_fsweep_labview_.dat", "CeCoIn5_3rd_8029_sam_12T_0.20K_60deg_changeT_fsweep_labview_.dat", "CeCoIn5_4th_8114_sam_12T_0.20K_30deg_changeT_fsweep_labview_.dat", "CeCoIn5_4th___40128__(042)__C(f)_12T_0.200K_45deg_changeT_ref_fromraw__labview_.dat", "CeCoIn5_4th___80128__(042)__C(f)_12T_0.200K_45deg_changeT_sam_fromraw__labview_.dat", "CeCoIn5_2nd_4050_12T_ref_0.22K_0deg_changeT_fsweep_labview_.dat", "CeCoIn5_2nd_4073_12T_ref_0.22K_90deg_changeT_fsweep_labview_.dat", "CeCoIn5_3rd_4030_ref_12T_0.24K_60deg_changeT_fsweep_labview_.dat", "CeCoIn5_3rd_8030_sam_12T_0.24K_60deg_changeT_fsweep_labview_.dat", "CeCoIn5_2nd_8074_12T_sam_0.249K_90deg_changeT_fsweep_labview_.dat", "CeCoIn5_4th_4115_ref_12T_0.25K_30deg_changeT_fsweep_labview_.dat", "CeCoIn5_2nd_8051_12T_sam_0.25K_0deg_changeT_fsweep_labview_.dat", "CeCoIn5_4th_8115_sam_12T_0.25K_30deg_changeT_fsweep_labview_.dat", "CeCoIn5_4th___40129__(043)__C(f)_12T_0.255K_45deg_changeT_ref_fromraw__labview_.dat", "CeCoIn5_4th___80129__(043)__C(f)_12T_0.255K_45deg_changeT_sam_fromraw__labview_.dat", "CeCoIn5_2nd_4074_12T_ref_0.27K_90deg_changeT_fsweep_labview_.dat", "CeCoIn5_2nd_4051_12T_ref_0.28K_0deg_changeT_fsweep_labview_.dat", "CeCoIn5_3rd_4031_ref_12T_0.287K_60deg_changeT_fsweep_labview_.dat", "CeCoIn5_3rd_8031_sam_12T_0.287K_60deg_changeT_fsweep_labview_.dat", "CeCoIn5_2nd_4094_6T_0.30K_90deg_ref_changeB_fsweep_labview_.dat", "CeCoIn5_4th_4116_ref_12T_0.30K_30deg_changeT_fsweep_labview_.dat", "CeCoIn5_2nd_8052_12T_sam_0.3K_0deg_changeT_fsweep_labview_.dat", "CeCoIn5_2nd_8075_12T_sam_0.300K_90deg_changeT_fsweep_labview_.dat", "CeCoIn5_2nd_8094_6T_0.30K_90deg_sam_changeB_fsweep_labview_.dat", "CeCoIn5_4th_8116_sam_12T_0.30K_30deg_changeT_fsweep_labview_.dat", "CeCoIn5_4th___40130__(044)__C(f)_12T_0.300K_45deg_changeT_ref_fromraw__labview_.dat", "CeCoIn5_4th___80130__(044)__C(f)_12T_0.300K_45deg_changeT_sam_fromraw__labview_.dat", "CeCoIn5_3rd_4032_ref_12T_0.33K_60deg_changeT_fsweep_labview_.dat", "CeCoIn5_2nd_4052_12T_ref_0.33K_0deg_changeT_fsweep_labview_.dat", "CeCoIn5_2nd_4075_12T_ref_0.33K_90deg_changeT_fsweep_labview_.dat", "CeCoIn5_3rd_8032_sam_12T_0.33K_60deg_changeT_fsweep_labview_.dat", "CeCoIn5_4th_4117_ref_12T_0.36K_30deg_changeT_fsweep_labview_.dat", "CeCoIn5_2nd_8053_12T_sam_0.360K_0deg_changeT_fsweep_labview_.dat", "CeCoIn5_2nd_8076_12T_sam_0.360K_90deg_changeT_fsweep_labview_.dat", "CeCoIn5_4th_8117_sam_12T_0.36K_30deg_changeT_fsweep_labview_.dat", "CeCoIn5_4th___40131__(045)__C(f)_12T_0.360K_45deg_changeT_ref_fromraw__labview_.dat", "CeCoIn5_4th___80131__(045)__C(f)_12T_0.360K_45deg_changeT_sam_fromraw__labview_.dat", "CeCoIn5_2nd_4076_12T_ref_0.39K_90deg_changeT_fsweep_labview_.dat", "CeCoIn5_2nd_4053_12T_ref_0.40K_0deg_changeT_fsweep_labview_.dat", "CeCoIn5_3rd_4033_ref_12T_0.43K_60deg_changeT_fsweep_labview_.dat", "CeCoIn5_4th_4118_ref_12T_0.43K_30deg_changeT_fsweep_labview_.dat", "CeCoIn5_3rd_8033_sam_12T_0.43K_60deg_changeT_fsweep_labview_.dat", "CeCoIn5_2nd_8054_12T_sam_0.430K_0deg_changeT_fsweep_labview_.dat", "CeCoIn5_2nd_8077_12T_sam_0.430K_90deg_changeT_fsweep_labview_.dat", "CeCoIn5_4th_8118_sam_12T_0.43K_30deg_changeT_fsweep_labview_.dat", "CeCoIn5_4th___40132__(046)__C(f)_12T_0.43K_45deg_changeT_ref_fromraw__labview_.dat", "CeCoIn5_4th___80132__(046)__C(f)_12T_0.43K_45deg_changeT_sam_fromraw__labview_.dat", "CeCoIn5_2nd_4054_12T_ref_0.48K_0deg_changeT_fsweep_labview_.dat", "CeCoIn5_2nd_4077_12T_ref_0.48K_90deg_changeT_fsweep_labview_.dat", "CeCoIn5_3rd_4034_ref_12T_0.51K_60deg_changeT_fsweep_labview_.dat", "CeCoIn5_3rd_8034_sam_12T_0.51K_60deg_changeT_fsweep_labview_.dat", "CeCoIn5_2nd_8055_12T_sam_0.512K_0deg_changeT_fsweep_labview_.dat", "CeCoIn5_2nd_8078_12T_sam_0.512K_90deg_changeT_fsweep_labview_.dat", "CeCoIn5_4th_4119_ref_12T_0.53K_30deg_changeT_fsweep_labview_.dat", "CeCoIn5_4th_8119_sam_12T_0.53K_30deg_changeT_fsweep_labview_.dat", "CeCoIn5_4th___40133__(047)__C(f)_12T_0.53K_45deg_changeT_ref_fromraw__labview_.dat", "CeCoIn5_4th___80133__(047)__C(f)_12T_0.53K_45deg_changeT_sam_fromraw__labview_.dat", "CeCoIn5_2nd_4055_12T_ref_0.58K_0deg_changeT_fsweep_labview_.dat", "CeCoIn5_2nd_4078_12T_ref_0.58K_90deg_changeT_fsweep_labview_.dat", "CeCoIn5_2nd_8056_12T_sam_0.61K_0deg_changeT_fsweep_labview_.dat", "CeCoIn5_2nd_8079_12T_sam_0.610K_90deg_changeT_fsweep_labview_.dat", "CeCoIn5_3rd_4035_ref_12T_0.62K_60deg_changeT_fsweep_labview_.dat", "CeCoIn5_4th_4120_ref_12T_0.62K_30deg_changeT_fsweep_labview_.dat", "CeCoIn5_3rd_8035_sam_12T_0.62K_60deg_changeT_fsweep_labview_.dat", "CeCoIn5_4th_8120_sam_12T_0.62K_30deg_changeT_fsweep_labview_.dat", "CeCoIn5_4th___40134__(048)__C(f)_12T_0.62K_45deg_changeT_ref_fromraw__labview_.dat", "CeCoIn5_4th___80134__(048)__C(f)_12T_0.62K_45deg_changeT_sam_fromraw__labview_.dat", "CeCoIn5_2nd_4108_0T_0.67K_90deg_ref_changeB_fsweep_labview_.dat", "CeCoIn5_2nd_8108_0T_0.67K_90deg_sam_changeB_fsweep_labview_.dat", "CeCoIn5_2nd_4056_12T_ref_0.68K_0deg_changeT_fsweep_labview_.dat", "CeCoIn5_2nd_4079_12T_ref_0.68K_90deg_changeT_fsweep_labview_.dat", "CeCoIn5_2nd_8057_12T_sam_0.81K_0deg_changeT_fsweep_labview_.dat", "CeCoIn5_2nd_8080_12T_sam_0.810K_90deg_changeT_fsweep_labview_.dat", "CeCoIn5_3rd_4036_ref_12T_0.83K_60deg_changeT_fsweep_labview_.dat", "CeCoIn5_4th_4121_ref_12T_0.83K_30deg_changeT_fsweep_labview_.dat", "CeCoIn5_3rd_8036_sam_12T_0.83K_60deg_changeT_fsweep_labview_.dat", "CeCoIn5_4th_8121_sam_12T_0.83K_30deg_changeT_fsweep_labview_.dat", "CeCoIn5_4th___40135__(049)__C(f)_12T_0.83K_45deg_changeT_ref_fromraw__labview_.dat", "CeCoIn5_4th___80135__(049)__C(f)_12T_0.83K_45deg_changeT_sam_fromraw__labview_.dat", "CeCoIn5_2nd_4057_12T_ref_0.91K_0deg_changeT_fsweep_labview_.dat", "CeCoIn5_2nd_4080_12T_ref_0.91K_90deg_changeT_fsweep_labview_.dat", "CeCoIn5_2nd_4107_0T_1.00K_90deg_ref_changeB_fsweep_labview_.dat", "CeCoIn5_2nd_8107_0T_1.00K_90deg_sam_changeB_fsweep_labview_.dat", "CeCoIn5_2nd_8081_12T_sam_1.1K_90deg_changeT_fsweep_labview_.dat", "CeCoIn5_2nd_8058_12T_sam_1.12K_0deg_changeT_fsweep_labview_.dat", "CeCoIn5_3rd_4037_ref_12T_1.13K_60deg_changeT_fsweep_labview_.dat", "CeCoIn5_4th_4122_ref_12T_1.13K_30deg_changeT_fsweep_labview_.dat", "CeCoIn5_3rd_8037_sam_12T_1.13K_60deg_changeT_fsweep_labview_.dat", "CeCoIn5_4th_8122_sam_12T_1.13K_30deg_changeT_fsweep_labview_.dat", "CeCoIn5_4th___40136__(050)__C(f)_12T_1.13K_45deg_changeT_ref_fromraw__labview_.dat", "CeCoIn5_4th___80136__(050)__C(f)_12T_1.13K_45deg_changeT_sam_fromraw__labview_.dat", "CeCoIn5_2nd_4058_12T_ref_1.23K_0deg_changeT_fsweep_labview_.dat", "CeCoIn5_2nd_4081_12T_ref_1.23K_90deg_changeT_fsweep_labview_.dat", "CeCoIn5_2nd_4106_0T_1.55K_90deg_ref_changeB_fsweep_labview_.dat", "CeCoIn5_2nd_8106_0T_1.55K_90deg_sam_changeB_fsweep_labview_.dat", "CeCoIn5_2nd_8059_12T_sam_1.8K_0deg_changeT_fsweep_labview_.dat", "CeCoIn5_2nd_8082_12T_sam_1.8K_90deg_changeT_fsweep_labview_.dat", "CeCoIn5_3rd_4038_ref_12T_1.90K_60deg_changeT_fsweep_labview_.dat", "CeCoIn5_4th_4123_ref_12T_1.90K_30deg_changeT_fsweep_labview_.dat", "CeCoIn5_3rd_8038_sam_12T_1.90K_60deg_changeT_fsweep_labview_.dat", "CeCoIn5_4th_8123_sam_12T_1.90K_30deg_changeT_fsweep_labview_.dat", "CeCoIn5_4th___40137__(051)__C(f)_12T_1.90K_45deg_changeT_ref_fromraw__labview_.dat", "CeCoIn5_4th___80137__(051)__C(f)_12T_1.90K_45deg_changeT_sam_fromraw__labview_.dat", "CeCoIn5_2nd_4059_12T_ref_1.97K_0deg_changeT_fsweep_labview_.dat", "CeCoIn5_2nd_4082_12T_ref_2.05K_90deg_changeT_fsweep_labview_.dat", "CeCoIn5_2nd_8060_12T_sam_3.0K_0deg_changeT_fsweep_labview_.dat", "CeCoIn5_2nd_8083_12T_sam_3.0K_90deg_changeT_fsweep_labview_.dat", "CeCoIn5_4th_4124_ref_12T_3.10K_30deg_changeT_fsweep_labview_.dat", "CeCoIn5_4th_8124_sam_12T_3.10K_30deg_changeT_fsweep_labview_.dat", "CeCoIn5_4th___40138__(052)__C(f)_12T_3.10K_45deg_changeT_ref_fromraw__labview_.dat", "CeCoIn5_4th___80138__(052)__C(f)_12T_3.10K_45deg_changeT_sam_fromraw__labview_.dat", "CeCoIn5_3rd_4039_ref_12T_3.15K_60deg_changeT_fsweep_labview_.dat", "CeCoIn5_3rd_8039_sam_12T_3.15K_60deg_changeT_fsweep_labview_.dat", "CeCoIn5_2nd_4060_12T_ref_3.19K_0deg_changeT_fsweep_labview_.dat", "CeCoIn5_2nd_4083_12T_ref_3.31K_90deg_changeT_fsweep_labview_.dat", "CeCoIn5_2nd_8061_12T_sam_5.5K_0deg_changeT_fsweep_labview_.dat", "CeCoIn5_3rd_4040_ref_12T_5.70K_60deg_changeT_fsweep_labview_.dat", "CeCoIn5_3rd_8040_sam_12T_5.70K_60deg_changeT_fsweep_labview_.dat", "CeCoIn5_2nd_8084_12T_sam_5.7K_90deg_changeT_fsweep_labview_.dat", "CeCoIn5_4th___40139__(053)__C(f)_12T_5.70K_45deg_changeT_ref_fromraw__labview_.dat", "CeCoIn5_4th___80139__(053)__C(f)_12T_5.70K_45deg_changeT_sam_fromraw__labview_.dat", "CeCoIn5_2nd_4061_12T_ref_5.82K_0deg_changeT_fsweep_labview_.dat", "CeCoIn5_2nd_4084_12T_ref_6.0K_90deg_changeT_fsweep_labview_.dat", "CeCoIn5_3rd_4041_ref_12T_7.87K_60deg_changeT_fsweep_labview_.dat", "CeCoIn5_3rd_8041_sam_12T_7.87K_60deg_changeT_fsweep_labview_.dat", "CeCoIn5_3rd_4042_ref_12T_9.80K_60deg_changeT_fsweep_labview_.dat", "CeCoIn5_3rd_8042_sam_12T_9.80K_60deg_changeT_fsweep_labview_.dat", "CeCoIn5_3rd_4043_ref_12T_12.36K_60deg_changeT_fsweep_labview_.dat", "CeCoIn5_3rd_8043_sam_12T_12.36K_60deg_changeT_fsweep_labview_.dat", "CeCoIn5_3rd_4044_ref_12T_14.80K_60deg_changeT_fsweep_labview_.dat", "CeCoIn5_3rd_8044_sam_12T_14.80K_60deg_changeT_fsweep_labview_.dat", "CeCoIn5_3rd_4045_ref_12T_16.42K_60deg_changeT_fsweep_labview_.dat", "CeCoIn5_3rd_8045_sam_12T_16.42K_60deg_changeT_fsweep_labview_.dat", "CeCoIn5_3rd_4046_ref_12T_18.04K_60deg_changeT_fsweep_labview_.dat", "CeCoIn5_3rd_8046_sam_12T_18.04K_60deg_changeT_fsweep_labview_.dat", "CeCoIn5_3rd_40047_ref_12T_19.60K_60deg_changeT_fsweep_labview_.dat", "CeCoIn5_3rd_80047_sam_12T_19.60K_60deg_changeT_fsweep_labview_.dat"]
  out "notes":string="------------\n\n/opt/new/Dropbox/desktop_data/Indium-nanocal-cell12-June2021/labview-ready-files\nIndium_June2021_*_ark.dat\n\n---------------------\n/opt/new/Dropbox/shared_AkashAndreas/paper-CeCoIn5/labviewreadydata\nCeCoIn5_*_labview_.dat\n--------------------------------\n\n  48 ->   <| \"ζ\"->  0.219100303741  , \"τ1\"-> 0.028643012604  , \"τS\"-> 0.279362928811  , \"τN\"-> 0.246156444058  , \"τC\"-> 0.001272401549  , \"κ0\"-> 0.000000000760  , \"mm1\"-> 0.000227975653  , \"mm2\"-> 0.014929571562  , \"mm3\"-> 0.655418694024  , \"T\"->  0.148000000000  , \"B\"-> 12.000000000000  , \"θ\"-> 0.000000000000  |>   , \r49 ->   <| \"ζ\"->  0.172530402516  , \"τ1\"-> 0.028151242536  , \"τS\"-> 0.147833386881  , \"τN\"-> 0.151615465647  , \"τC\"-> 0.001078987959  , \"κ0\"-> 0.000000001040  , \"mm1\"-> 0.000157922197  , \"mm2\"-> 0.013374167913  , \"mm3\"-> 0.366811023972  , \"T\"->  0.179000000000  , \"B\"-> 12.000000000000  , \"θ\"-> 0.000000000000  |>   , \r50 ->   <| \"ζ\"->  0.133463068512  , \"τ1\"-> 0.025720252342  , \"τS\"-> 0.123146502099  , \"τN\"-> 0.097478248186  , \"τC\"-> 0.001335222055  , \"κ0\"-> 0.000000001204  , \"mm1\"-> 0.000155896243  , \"mm2\"-> 0.013755191011  , \"mm3\"-> 0.263214393590  , \"T\"->  0.197000000000  , \"B\"-> 12.000000000000  , \"θ\"-> 0.000000000000  |>   , \r51 ->   <| \"ζ\"->  0.081993362741  , \"τ1\"-> 0.028064095915  , \"τS\"-> 0.091433392476  , \"τN\"-> 0.030443971714  , \"τC\"-> 0.001450504959  , \"κ0\"-> 0.000000001536  , \"mm1\"-> 0.000108446090  , \"mm2\"-> 0.019905820843  , \"mm3\"-> 0.141370833064  , \"T\"->  0.250000000000  , \"B\"-> 12.000000000000  , \"θ\"-> 0.000000000000  |>   , \r52 ->   <| \"ζ\"->  0.054088186012  , \"τ1\"-> 0.023838802615  , \"τS\"-> 0.069079396629  , \"τN\"-> 0.016435267456  , \"τC\"-> 0.002025071743  , \"κ0\"-> 0.000000001955  , \"mm1\"-> 0.000101234646  , \"mm2\"-> 0.018244822177  , \"mm3\"-> 0.097657814678  , \"T\"->  0.300000000000  , \"B\"-> 12.000000000000  , \"θ\"-> 0.000000000000  |>   , \r53 ->   <| \"ζ\"->  0.039314966212  , \"τ1\"-> 0.020712803909  , \"τS\"-> 0.055413767550  , \"τN\"-> 0.008474403424  , \"τC\"-> 0.002674063387  , \"κ0\"-> 0.000000002415  , \"mm1\"-> 0.000096818147  , \"mm2\"-> 0.017190811405  , \"mm3\"-> 0.072499170001  , \"T\"->  0.360000000000  , \"B\"-> 12.000000000000  , \"θ\"-> 0.000000000000  |>   , \r54 ->   <| \"ζ\"->  0.031945976845  , \"τ1\"-> 0.019000922826  , \"τS\"-> 0.045624146388  , \"τN\"-> 0.005314716063  , \"τC\"-> 0.002488383471  , \"κ0\"-> 0.000000002954  , \"mm1\"-> 0.000073272643  , \"mm2\"-> 0.016306894362  , \"mm3\"-> 0.057675293464  , \"T\"->  0.430000000000  , \"B\"-> 12.000000000000  , \"θ\"-> 0.000000000000  |>   , \r55 ->   <| \"ζ\"->  0.023031239946  , \"τ1\"-> 0.018268814012  , \"τS\"-> 0.037269400776  , \"τN\"-> 0.002696792890  , \"τC\"-> 0.003257395394  , \"κ0\"-> 0.000000003720  , \"mm1\"-> 0.000067670174  , \"mm2\"-> 0.016445281937  , \"mm3\"-> 0.045899921957  , \"T\"->  0.512000000000  , \"B\"-> 12.000000000000  , \"θ\"-> 0.000000000000  |>   , \r56 ->   <| \"ζ\"->  0.019920170845  , \"τ1\"-> 0.016368892412  , \"τS\"-> 0.030579536580  , \"τN\"-> 0.001736017565  , \"τC\"-> 0.004971418152  , \"κ0\"-> 0.000000004410  , \"mm1\"-> 0.000083939556  , \"mm2\"-> 0.015095997595  , \"mm3\"-> 0.039119658918  , \"T\"->  0.610000000000  , \"B\"-> 12.000000000000  , \"θ\"-> 0.000000000000  |>   , \r57 ->   <| \"ζ\"->  0.017558473054  , \"τ1\"-> 0.014545104284  , \"τS\"-> 0.022979681288  , \"τN\"-> 0.000840829385  , \"τC\"-> 0.005228030240  , \"κ0\"-> 0.000000006068  , \"mm1\"-> 0.000073916527  , \"mm2\"-> 0.013750428362  , \"mm3\"-> 0.030187552103  , \"T\"->  0.810000000000  , \"B\"-> 12.000000000000  , \"θ\"-> 0.000000000000  |>   , \r58 ->   <| \"ζ\"->  0.011916480594  , \"τ1\"-> 0.012551282481  , \"τS\"-> 0.018233218660  , \"τN\"-> 0.000345702746  , \"τC\"-> 0.004699451527  , \"κ0\"-> 0.000000008451  , \"mm1\"-> 0.000044190864  , \"mm2\"-> 0.012162820727  , \"mm3\"-> 0.023844039179  , \"T\"->  1.120000000000  , \"B\"-> 12.000000000000  , \"θ\"-> 0.000000000000  |>   , \r59 ->   <| \"ζ\"->  0.012831327568  , \"τ1\"-> 0.013315909415  , \"τS\"-> 0.012590836847  , \"τN\"-> 0.000065003013  , \"τC\"-> 0.005276356243  , \"κ0\"-> 0.000000013610  , \"mm1\"-> 0.000047406274  , \"mm2\"-> 0.013137605540  , \"mm3\"-> 0.018225484932  , \"T\"->  1.800000000000  , \"B\"-> 12.000000000000  , \"θ\"-> 0.000000000000  |>   , \r60 ->   <| \"ζ\"->  0.019774146838  , \"τ1\"-> 0.013257273421  , \"τS\"-> 0.007064131508  , \"τN\"-> 0.000028000819  , \"τC\"-> 0.006942241845  , \"κ0\"-> 0.000000023477  , \"mm1\"-> 0.000068886863  , \"mm2\"-> 0.012935419574  , \"mm3\"-> 0.014427582022  , \"T\"->  3.000000000000  , \"B\"-> 12.000000000000  , \"θ\"-> 0.000000000000  |>   , \r61 ->   <| \"ζ\"->  0.029251354442  , \"τ1\"-> 0.014634751206  , \"τS\"-> 0.003873958746  , \"τN\"-> 0.000007000487  , \"τC\"-> 0.006827504775  , \"κ0\"-> 0.000000056438  , \"mm1\"-> 0.000072018576  , \"mm2\"-> 0.010723236476  , \"mm3\"-> 0.014661483476  , \"T\"->  5.500000000000  , \"B\"-> 12.000000000000  , \"θ\"-> 0.000000000000  |>   , \r70 ->   <| \"ζ\"->  0.166131699293  , \"τ1\"-> 0.072775930308  , \"τS\"-> 0.042465819987  , \"τN\"-> 0.161702990281  , \"τC\"-> 0.001278548133  , \"κ0\"-> 0.000000001029  , \"mm1\"-> 0.000178150965  , \"mm2\"-> 0.012296129795  , \"mm3\"-> 0.299667919341  , \"T\"->  0.179000000000  , \"B\"-> 12.000000000000  , \"θ\"-> 90.000000000000  |>   , \r71 ->   <| \"ζ\"->  0.300863384227  , \"τ1\"-> 0.104924004009  , \"τS\"-> 0.071070599729  , \"τN\"-> 0.992887187112  , \"τC\"-> 0.001721587800  , \"κ0\"-> 0.000000000548  , \"mm1\"-> 0.000392216822  , \"mm2\"-> 0.006637384427  , \"mm3\"-> 1.483679717825  , \"T\"->  0.120000000000  , \"B\"-> 12.000000000000  , \"θ\"-> 90.000000000000  |>   , \r72 ->   <| \"ζ\"->  0.222191124978  , \"τ1\"-> 0.096157808510  , \"τS\"-> 0.068016409177  , \"τN\"-> 0.365932480375  , \"τC\"-> 0.001342124138  , \"κ0\"-> 0.000000000769  , \"mm1\"-> 0.000240761160  , \"mm2\"-> 0.013184061080  , \"mm3\"-> 0.614443591912  , \"T\"->  0.148000000000  , \"B\"-> 12.000000000000  , \"θ\"-> 90.000000000000  |>   , \r73 ->   <| \"ζ\"->  0.136299067728  , \"τ1\"-> 0.070555788073  , \"τS\"-> 0.041728112583  , \"τN\"-> 0.122673380524  , \"τC\"-> 0.001576035942  , \"κ0\"-> 0.000000001215  , \"mm1\"-> 0.000183611814  , \"mm2\"-> 0.014077355758  , \"mm3\"-> 0.244680119794  , \"T\"->  0.197000000000  , \"B\"-> 12.000000000000  , \"θ\"-> 90.000000000000  |>   , \r74 ->   <| \"ζ\"->  0.083818989463  , \"τ1\"-> 0.054019568165  , \"τS\"-> 0.033709166928  , \"τN\"-> 0.048192327645  , \"τC\"-> 0.001574712191  , \"κ0\"-> 0.000000001532  , \"mm1\"-> 0.000117096712  , \"mm2\"-> 0.016005996433  , \"mm3\"-> 0.128237582295  , \"T\"->  0.249000000000  , \"B\"-> 12.000000000000  , \"θ\"-> 90.000000000000  |>   , \r75 ->   <| \"ζ\"->  0.057938569833  , \"τ1\"-> 0.045244527663  , \"τS\"-> 0.029709028064  , \"τN\"-> 0.023577376257  , \"τC\"-> 0.002006607539  , \"κ0\"-> 0.000000001948  , 
